vi "Init.vi"(10 "Port":u32, 11 "IP":string) -> (0 "error out":errorcluster, 3 "DB_API.lvclass 2":refnum<class "DB_API.lvclass">)   [LabVIEW 2024, in "DB_API.lvclass"]
uses:
  DB_API.lvclass
  DB_API.lvclass/DB_API.ctl
  <vilib>/httpClient/LabVIEWHTTPClient.lvlib
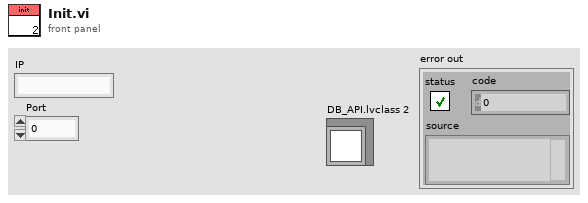
[diagram p1: front panel]
types:
  T1 = typedef "LabVIEWHTTPClient.lvlib/ClientHandle.ctl" = refnum<k1>
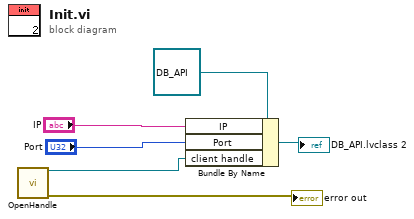
[diagram p0: block diagram]
diagram:
  n1 = call <vilib>:"OpenHandle.vi"() -> ("client handle out"=w5:T1, "error out"=→"error out":errorcluster)  [unwired: 14 in]
  n2 = Bundle By Name(cluster=refnum<class "DB_API.lvclass"> refnum ("DB_API.lvclass"), "IP"="IP", "Port"="Port", "client handle"=w5) -> (→"DB_API.lvclass 2":refnum<class "DB_API.lvclass">)
